vi "Read X-Axis.vi"(6 "Maximum Time (10000 ms)":u32=10000, 8 "error in (no error)":errorcluster, 9 "Select Trace (1: 1)":u16(ring)=1 items=["1"=1, "2"=2, "3"=3, "4"=4, "5"=5, "6"=6, "7"=7, "8"=8], 10 "Measurement Type (6: Phase Noise)":u16(ring)=6 items=["AM Noise"=1, "Baseband Noise"=2, "Freq/Power"=3, "Spectrum"=4, "Transient"=5, "Phase Noise"=6, "User"=7], 11 "VISA resource name":refnum<visa-resource-name>) -> (0 "error out":errorcluster, 2 "Measurements":dbl[](array[numeric]) format="%^#_9g", 3 "VISA resource name out":refnum<visa-resource-name>)   [LabVIEW 2011, in "Agilent E5052X.lvlib"]
doc: "Reads X-axis trace data from the instrument."
uses:
  Agilent E5052X.lvlib
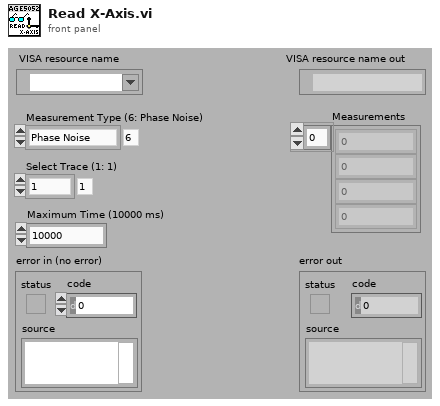
[diagram p1: front panel]
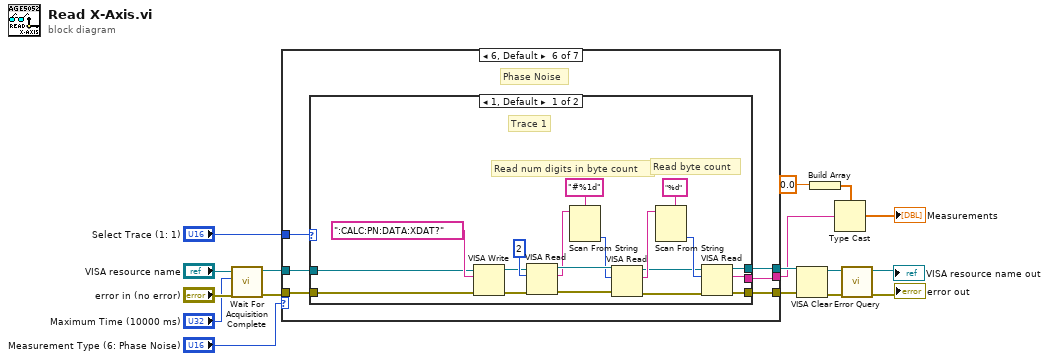
[diagram p0: block diagram]
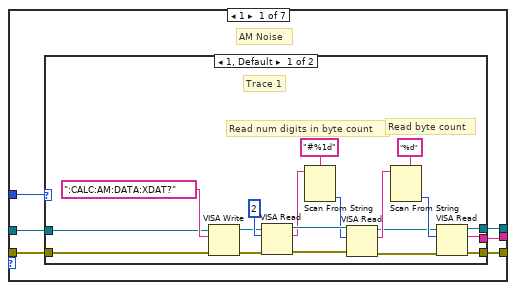
[diagram p2: hidden frame]
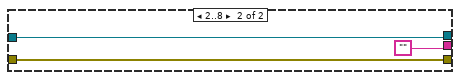
[diagram p3: hidden frame]
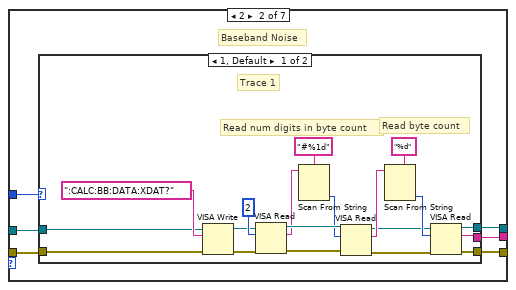
[diagram p4: hidden frame]
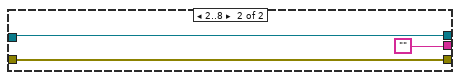
[diagram p5: hidden frame]
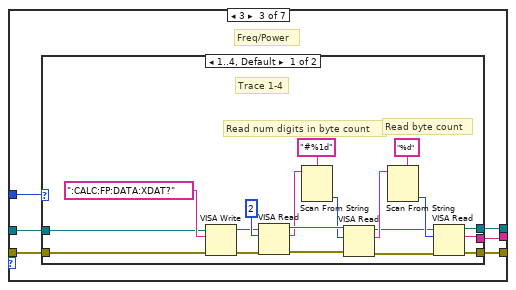
[diagram p6: hidden frame]
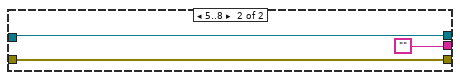
[diagram p7: hidden frame]
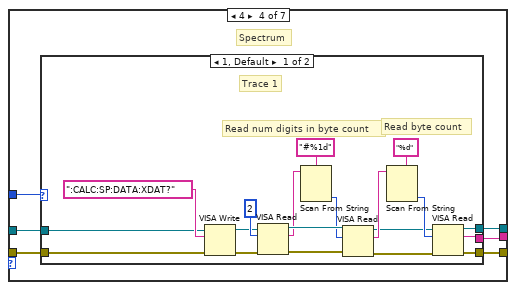
[diagram p8: hidden frame]
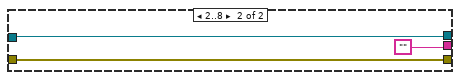
[diagram p9: hidden frame]
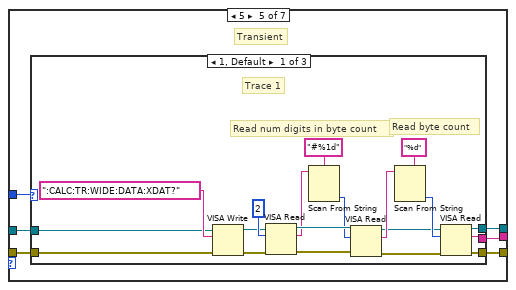
[diagram p10: hidden frame]
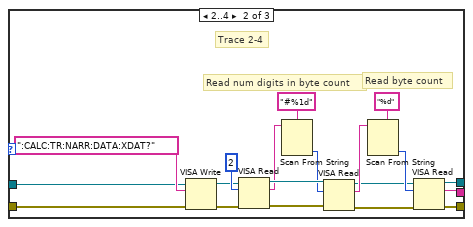
[diagram p11: hidden frame]
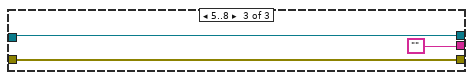
[diagram p12: hidden frame]
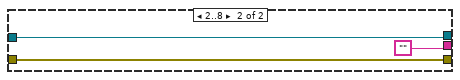
[diagram p13: hidden frame]
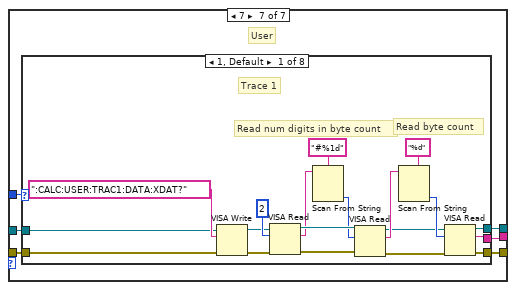
[diagram p14: hidden frame]
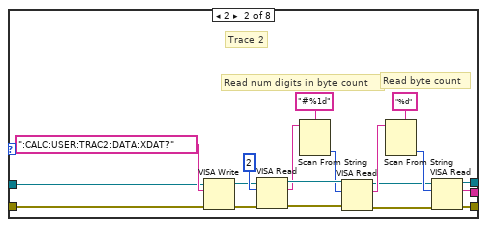
[diagram p15: hidden frame]
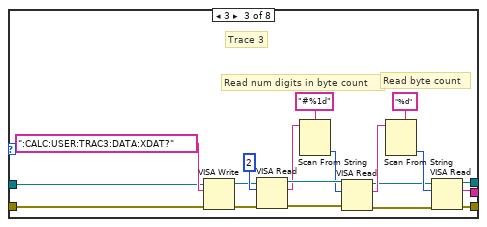
[diagram p16: hidden frame]
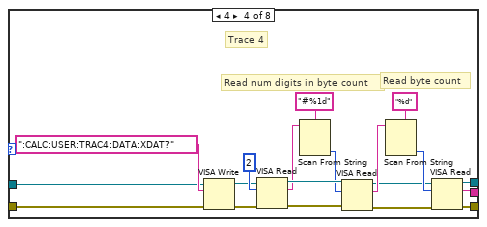
[diagram p17: hidden frame]
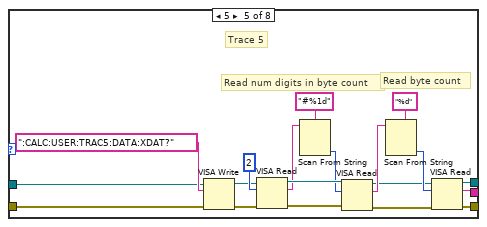
[diagram p18: hidden frame]
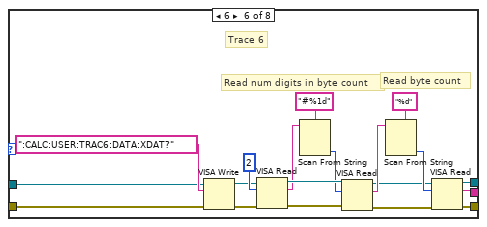
[diagram p19: hidden frame]
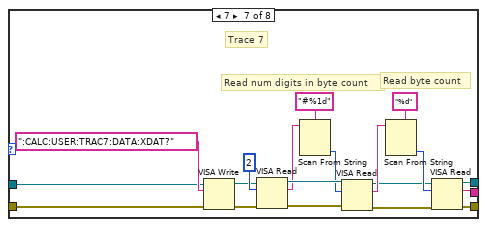
[diagram p20: hidden frame]
diagram:
  n1 = call "Wait For Acquisition Complete.vi"("error in (no error)"="error in (no error)", "Maximum Time (10000)"="Maximum Time (10000 ms)", "VISA resource name"="VISA resource name") -> ("error out"=w11:errorcluster, "VISA resource name out"=w10:refnum<visa-resource-name>)  [unwired: 7 in]
  n2 = case shown="6, Default" "Measurement Type (6: Phase Noise)" {
    tunnel: w10 -> [w22 w50 w78 w106 w134 w181 w209]
    tunnel: w11 -> [w21 w49 w77 w105 w133 w180 w208]
    tunnel: "Select Trace (1: 1)" -> [w23 w51 w79 w107 w135 w182 w210]
    tunnel: [w20 w48 w76 w104 w132 w179 w207] -> w13
    tunnel: [w19 w46 w74 w102 w130 w177 w205] -> w12
    tunnel: [w18 w47 w75 w103 w131 w178 w206] -> w2
    frame 1 {
      # "AM Noise"
      n3 = case shown="1, Default" w23 {
        tunnel: w22 -> [w41 w45]
        tunnel: w21 -> [w40 w44]
        tunnel: [w26 w45] -> w20
        tunnel: [w25 w44] -> w19
        tunnel: [w24 ""] -> w18
        frame 1, Default {
          # "Read num digits in byte count"
          # "Read byte count"
          # "Trace 1"
          n4 = VISA Write(VISA resource name=w41, write buffer=":CALC:AM:DATA:XDAT?" ("format string"), error in (no error)=w40) -> (VISA resource name out=w30:refnum<visa-resource-name>, error out=w29:errorcluster)  [unwired: 1 out]
          n5 = VISA Read(VISA resource name=w30, byte count=u32 2, error in (no error)=w29) -> (VISA resource name out=w36:refnum<visa-resource-name>, read buffer=w32:string, error out=w37:errorcluster)  [unwired: 1 out]
          n6 = Scan From String(format string="#%1d", input string=w32) -> (output 1=w35:i32)  [unwired: 3 in, 3 out]
          n7 = VISA Read(VISA resource name=w36, byte count=w35, error in (no error)=w37) -> (VISA resource name out=w28:refnum<visa-resource-name>, read buffer=w34:string, error out=w27:errorcluster)  [unwired: 1 out]
          n8 = Scan From String(format string="%d", input string=w34) -> (output 1=w31:i32)  [unwired: 3 in, 3 out]
          n9 = VISA Read(VISA resource name=w28, byte count=w31, error in (no error)=w27) -> (VISA resource name out=w26:refnum<visa-resource-name>, read buffer=w24:string, error out=w25:errorcluster)  [unwired: 1 out]
        }
        frame 2..8 {
        }
      }
    }
    frame 2 {
      # "Baseband Noise"
      n10 = case shown="1, Default" w51 {
        tunnel: w50 -> [w69 w73]
        tunnel: w49 -> [w68 w72]
        tunnel: [w54 w73] -> w48
        tunnel: [w53 w72] -> w46
        tunnel: [w52 ""] -> w47
        frame 1, Default {
          # "Read num digits in byte count"
          # "Read byte count"
          # "Trace 1"
          n11 = VISA Write(VISA resource name=w69, write buffer=":CALC:BB:DATA:XDAT?" ("format string"), error in (no error)=w68) -> (VISA resource name out=w58:refnum<visa-resource-name>, error out=w57:errorcluster)  [unwired: 1 out]
          n12 = VISA Read(VISA resource name=w58, byte count=u32 2, error in (no error)=w57) -> (VISA resource name out=w64:refnum<visa-resource-name>, read buffer=w60:string, error out=w65:errorcluster)  [unwired: 1 out]
          n13 = Scan From String(format string="#%1d", input string=w60) -> (output 1=w63:i32)  [unwired: 3 in, 3 out]
          n14 = VISA Read(VISA resource name=w64, byte count=w63, error in (no error)=w65) -> (VISA resource name out=w56:refnum<visa-resource-name>, read buffer=w62:string, error out=w55:errorcluster)  [unwired: 1 out]
          n15 = Scan From String(format string="%d", input string=w62) -> (output 1=w59:i32)  [unwired: 3 in, 3 out]
          n16 = VISA Read(VISA resource name=w56, byte count=w59, error in (no error)=w55) -> (VISA resource name out=w54:refnum<visa-resource-name>, read buffer=w52:string, error out=w53:errorcluster)  [unwired: 1 out]
        }
        frame 2..8 {
        }
      }
    }
    frame 3 {
      # "Freq/Power"
      n17 = case shown="1..4, Default" w79 {
        tunnel: w78 -> [w97 w101]
        tunnel: w77 -> [w96 w100]
        tunnel: [w82 w101] -> w76
        tunnel: [w81 w100] -> w74
        tunnel: [w80 ""] -> w75
        frame 1..4, Default {
          # "Trace 1-4"
          # "Read num digits in byte count"
          # "Read byte count"
          n18 = VISA Write(VISA resource name=w97, write buffer=":CALC:FP:DATA:XDAT?" ("format string"), error in (no error)=w96) -> (VISA resource name out=w86:refnum<visa-resource-name>, error out=w85:errorcluster)  [unwired: 1 out]
          n19 = VISA Read(VISA resource name=w86, byte count=u32 2, error in (no error)=w85) -> (VISA resource name out=w92:refnum<visa-resource-name>, read buffer=w88:string, error out=w93:errorcluster)  [unwired: 1 out]
          n20 = Scan From String(format string="#%1d", input string=w88) -> (output 1=w91:i32)  [unwired: 3 in, 3 out]
          n21 = VISA Read(VISA resource name=w92, byte count=w91, error in (no error)=w93) -> (VISA resource name out=w84:refnum<visa-resource-name>, read buffer=w90:string, error out=w83:errorcluster)  [unwired: 1 out]
          n22 = Scan From String(format string="%d", input string=w90) -> (output 1=w87:i32)  [unwired: 3 in, 3 out]
          n23 = VISA Read(VISA resource name=w84, byte count=w87, error in (no error)=w83) -> (VISA resource name out=w82:refnum<visa-resource-name>, read buffer=w80:string, error out=w81:errorcluster)  [unwired: 1 out]
        }
        frame 5..8 {
        }
      }
    }
    frame 4 {
      # "Spectrum"
      n24 = case shown="1, Default" w107 {
        tunnel: w106 -> [w125 w127]
        tunnel: w105 -> [w124 w129]
        tunnel: [w110 w127] -> w104
        tunnel: [w109 w129] -> w102
        tunnel: [w108 ""] -> w103
        frame 1, Default {
          # "Read num digits in byte count"
          # "Read byte count"
          # "Trace 1"
          n25 = VISA Write(VISA resource name=w125, write buffer=":CALC:SP:DATA:XDAT?" ("format string"), error in (no error)=w124) -> (VISA resource name out=w114:refnum<visa-resource-name>, error out=w113:errorcluster)  [unwired: 1 out]
          n26 = VISA Read(VISA resource name=w114, byte count=u32 2, error in (no error)=w113) -> (VISA resource name out=w120:refnum<visa-resource-name>, read buffer=w116:string, error out=w121:errorcluster)  [unwired: 1 out]
          n27 = Scan From String(format string="#%1d", input string=w116) -> (output 1=w119:i32)  [unwired: 3 in, 3 out]
          n28 = VISA Read(VISA resource name=w120, byte count=w119, error in (no error)=w121) -> (VISA resource name out=w112:refnum<visa-resource-name>, read buffer=w118:string, error out=w111:errorcluster)  [unwired: 1 out]
          n29 = Scan From String(format string="%d", input string=w118) -> (output 1=w115:i32)  [unwired: 3 in, 3 out]
          n30 = VISA Read(VISA resource name=w112, byte count=w115, error in (no error)=w111) -> (VISA resource name out=w110:refnum<visa-resource-name>, read buffer=w108:string, error out=w109:errorcluster)  [unwired: 1 out]
        }
        frame 2..8 {
        }
      }
    }
    frame 5 {
      # "Transient"
      n31 = case shown="1, Default" w135 {
        tunnel: w134 -> [w140 w172 w176]
        tunnel: w133 -> [w139 w171 w175]
        tunnel: [w138 w157 w176] -> w132
        tunnel: [w136 w156 w175] -> w130
        tunnel: [w137 w155 ""] -> w131
        frame 1, Default {
          # "Trace 1"
          # "Read num digits in byte count"
          # "Read byte count"
          n32 = VISA Write(VISA resource name=w140, write buffer=":CALC:TR:WIDE:DATA:XDAT?" ("format string"), error in (no error)=w139) -> (VISA resource name out=w144:refnum<visa-resource-name>, error out=w143:errorcluster)  [unwired: 1 out]
          n33 = VISA Read(VISA resource name=w144, byte count=u32 2, error in (no error)=w143) -> (VISA resource name out=w150:refnum<visa-resource-name>, read buffer=w146:string, error out=w151:errorcluster)  [unwired: 1 out]
          n34 = Scan From String(format string="#%1d", input string=w146) -> (output 1=w149:i32)  [unwired: 3 in, 3 out]
          n35 = VISA Read(VISA resource name=w150, byte count=w149, error in (no error)=w151) -> (VISA resource name out=w142:refnum<visa-resource-name>, read buffer=w148:string, error out=w141:errorcluster)  [unwired: 1 out]
          n36 = Scan From String(format string="%d", input string=w148) -> (output 1=w145:i32)  [unwired: 3 in, 3 out]
          n37 = VISA Read(VISA resource name=w142, byte count=w145, error in (no error)=w141) -> (VISA resource name out=w138:refnum<visa-resource-name>, read buffer=w137:string, error out=w136:errorcluster)  [unwired: 1 out]
        }
        frame 2..4 {
          # "Trace 2-4"
          # "Read num digits in byte count"
          # "Read byte count"
          n38 = VISA Write(VISA resource name=w172, write buffer=":CALC:TR:NARR:DATA:XDAT?" ("format string"), error in (no error)=w171) -> (VISA resource name out=w161:refnum<visa-resource-name>, error out=w160:errorcluster)  [unwired: 1 out]
          n39 = VISA Read(VISA resource name=w161, byte count=u32 2, error in (no error)=w160) -> (VISA resource name out=w167:refnum<visa-resource-name>, read buffer=w163:string, error out=w168:errorcluster)  [unwired: 1 out]
          n40 = Scan From String(format string="#%1d", input string=w163) -> (output 1=w166:i32)  [unwired: 3 in, 3 out]
          n41 = VISA Read(VISA resource name=w167, byte count=w166, error in (no error)=w168) -> (VISA resource name out=w159:refnum<visa-resource-name>, read buffer=w165:string, error out=w158:errorcluster)  [unwired: 1 out]
          n42 = Scan From String(format string="%d", input string=w165) -> (output 1=w162:i32)  [unwired: 3 in, 3 out]
          n43 = VISA Read(VISA resource name=w159, byte count=w162, error in (no error)=w158) -> (VISA resource name out=w157:refnum<visa-resource-name>, read buffer=w155:string, error out=w156:errorcluster)  [unwired: 1 out]
        }
        frame 5..8 {
        }
      }
    }
    frame 6, Default {
      # "Phase Noise"
      n44 = case shown="1, Default" w182 {
        tunnel: w181 -> [w200 w204]
        tunnel: w180 -> [w199 w203]
        tunnel: [w185 w204] -> w179
        tunnel: [w184 w203] -> w177
        tunnel: [w183 ""] -> w178
        frame 1, Default {
          # "Read num digits in byte count"
          # "Read byte count"
          # "Trace 1"
          n45 = VISA Write(VISA resource name=w200, write buffer=":CALC:PN:DATA:XDAT?" ("format string"), error in (no error)=w199) -> (VISA resource name out=w189:refnum<visa-resource-name>, error out=w188:errorcluster)  [unwired: 1 out]
          n46 = VISA Read(VISA resource name=w189, byte count=u32 2, error in (no error)=w188) -> (VISA resource name out=w195:refnum<visa-resource-name>, read buffer=w191:string, error out=w196:errorcluster)  [unwired: 1 out]
          n47 = Scan From String(format string="#%1d", input string=w191) -> (output 1=w194:i32)  [unwired: 3 in, 3 out]
          n48 = VISA Read(VISA resource name=w195, byte count=w194, error in (no error)=w196) -> (VISA resource name out=w187:refnum<visa-resource-name>, read buffer=w193:string, error out=w186:errorcluster)  [unwired: 1 out]
          n49 = Scan From String(format string="%d", input string=w193) -> (output 1=w190:i32)  [unwired: 3 in, 3 out]
          n50 = VISA Read(VISA resource name=w187, byte count=w190, error in (no error)=w186) -> (VISA resource name out=w185:refnum<visa-resource-name>, read buffer=w183:string, error out=w184:errorcluster)  [unwired: 1 out]
        }
        frame 2..8 {
        }
      }
    }
    frame 7 {
      # "User"
      n51 = case shown="1, Default" w210 {
        tunnel: w209 -> [w228 w247 w266 w285 w304 w323 w342 w361]
        tunnel: w208 -> [w227 w246 w265 w284 w303 w322 w341 w360]
        tunnel: [w213 w232 w251 w270 w289 w308 w327 w346] -> w207
        tunnel: [w212 w231 w250 w269 w288 w307 w326 w345] -> w205
        tunnel: [w211 w230 w249 w268 w287 w306 w325 w344] -> w206
        frame 1, Default {
          # "Trace 1"
          # "Read num digits in byte count"
          # "Read byte count"
          n52 = VISA Write(VISA resource name=w228, write buffer=":CALC:USER:TRAC1:DATA:XDAT?" ("format string"), error in (no error)=w227) -> (VISA resource name out=w217:refnum<visa-resource-name>, error out=w216:errorcluster)  [unwired: 1 out]
          n53 = VISA Read(VISA resource name=w217, byte count=u32 2, error in (no error)=w216) -> (VISA resource name out=w223:refnum<visa-resource-name>, read buffer=w219:string, error out=w224:errorcluster)  [unwired: 1 out]
          n54 = Scan From String(format string="#%1d", input string=w219) -> (output 1=w222:i32)  [unwired: 3 in, 3 out]
          n55 = VISA Read(VISA resource name=w223, byte count=w222, error in (no error)=w224) -> (VISA resource name out=w215:refnum<visa-resource-name>, read buffer=w221:string, error out=w214:errorcluster)  [unwired: 1 out]
          n56 = Scan From String(format string="%d", input string=w221) -> (output 1=w218:i32)  [unwired: 3 in, 3 out]
          n57 = VISA Read(VISA resource name=w215, byte count=w218, error in (no error)=w214) -> (VISA resource name out=w213:refnum<visa-resource-name>, read buffer=w211:string, error out=w212:errorcluster)  [unwired: 1 out]
        }
        frame 2 {
          # "Trace 2"
          # "Read num digits in byte count"
          # "Read byte count"
          n58 = VISA Write(VISA resource name=w247, write buffer=":CALC:USER:TRAC2:DATA:XDAT?" ("format string"), error in (no error)=w246) -> (VISA resource name out=w236:refnum<visa-resource-name>, error out=w235:errorcluster)  [unwired: 1 out]
          n59 = VISA Read(VISA resource name=w236, byte count=u32 2, error in (no error)=w235) -> (VISA resource name out=w242:refnum<visa-resource-name>, read buffer=w238:string, error out=w243:errorcluster)  [unwired: 1 out]
          n60 = Scan From String(format string="#%1d", input string=w238) -> (output 1=w241:i32)  [unwired: 3 in, 3 out]
          n61 = VISA Read(VISA resource name=w242, byte count=w241, error in (no error)=w243) -> (VISA resource name out=w234:refnum<visa-resource-name>, read buffer=w240:string, error out=w233:errorcluster)  [unwired: 1 out]
          n62 = Scan From String(format string="%d", input string=w240) -> (output 1=w237:i32)  [unwired: 3 in, 3 out]
          n63 = VISA Read(VISA resource name=w234, byte count=w237, error in (no error)=w233) -> (VISA resource name out=w232:refnum<visa-resource-name>, read buffer=w230:string, error out=w231:errorcluster)  [unwired: 1 out]
        }
        frame 3 {
          # "Trace 3"
          # "Read num digits in byte count"
          # "Read byte count"
          n64 = VISA Write(VISA resource name=w266, write buffer=":CALC:USER:TRAC3:DATA:XDAT?" ("format string"), error in (no error)=w265) -> (VISA resource name out=w255:refnum<visa-resource-name>, error out=w254:errorcluster)  [unwired: 1 out]
          n65 = VISA Read(VISA resource name=w255, byte count=u32 2, error in (no error)=w254) -> (VISA resource name out=w261:refnum<visa-resource-name>, read buffer=w257:string, error out=w262:errorcluster)  [unwired: 1 out]
          n66 = Scan From String(format string="#%1d", input string=w257) -> (output 1=w260:i32)  [unwired: 3 in, 3 out]
          n67 = VISA Read(VISA resource name=w261, byte count=w260, error in (no error)=w262) -> (VISA resource name out=w253:refnum<visa-resource-name>, read buffer=w259:string, error out=w252:errorcluster)  [unwired: 1 out]
          n68 = Scan From String(format string="%d", input string=w259) -> (output 1=w256:i32)  [unwired: 3 in, 3 out]
          n69 = VISA Read(VISA resource name=w253, byte count=w256, error in (no error)=w252) -> (VISA resource name out=w251:refnum<visa-resource-name>, read buffer=w249:string, error out=w250:errorcluster)  [unwired: 1 out]
        }
        frame 4 {
          # "Trace 4"
          # "Read num digits in byte count"
          # "Read byte count"
          n70 = VISA Write(VISA resource name=w285, write buffer=":CALC:USER:TRAC4:DATA:XDAT?" ("format string"), error in (no error)=w284) -> (VISA resource name out=w274:refnum<visa-resource-name>, error out=w273:errorcluster)  [unwired: 1 out]
          n71 = VISA Read(VISA resource name=w274, byte count=u32 2, error in (no error)=w273) -> (VISA resource name out=w280:refnum<visa-resource-name>, read buffer=w276:string, error out=w281:errorcluster)  [unwired: 1 out]
          n72 = Scan From String(format string="#%1d", input string=w276) -> (output 1=w279:i32)  [unwired: 3 in, 3 out]
          n73 = VISA Read(VISA resource name=w280, byte count=w279, error in (no error)=w281) -> (VISA resource name out=w272:refnum<visa-resource-name>, read buffer=w278:string, error out=w271:errorcluster)  [unwired: 1 out]
          n74 = Scan From String(format string="%d", input string=w278) -> (output 1=w275:i32)  [unwired: 3 in, 3 out]
          n75 = VISA Read(VISA resource name=w272, byte count=w275, error in (no error)=w271) -> (VISA resource name out=w270:refnum<visa-resource-name>, read buffer=w268:string, error out=w269:errorcluster)  [unwired: 1 out]
        }
        frame 5 {
          # "Trace 5"
          # "Read num digits in byte count"
          # "Read byte count"
          n76 = VISA Write(VISA resource name=w304, write buffer=":CALC:USER:TRAC5:DATA:XDAT?" ("format string"), error in (no error)=w303) -> (VISA resource name out=w293:refnum<visa-resource-name>, error out=w292:errorcluster)  [unwired: 1 out]
          n77 = VISA Read(VISA resource name=w293, byte count=u32 2, error in (no error)=w292) -> (VISA resource name out=w299:refnum<visa-resource-name>, read buffer=w295:string, error out=w300:errorcluster)  [unwired: 1 out]
          n78 = Scan From String(format string="#%1d", input string=w295) -> (output 1=w298:i32)  [unwired: 3 in, 3 out]
          n79 = VISA Read(VISA resource name=w299, byte count=w298, error in (no error)=w300) -> (VISA resource name out=w291:refnum<visa-resource-name>, read buffer=w297:string, error out=w290:errorcluster)  [unwired: 1 out]
          n80 = Scan From String(format string="%d", input string=w297) -> (output 1=w294:i32)  [unwired: 3 in, 3 out]
          n81 = VISA Read(VISA resource name=w291, byte count=w294, error in (no error)=w290) -> (VISA resource name out=w289:refnum<visa-resource-name>, read buffer=w287:string, error out=w288:errorcluster)  [unwired: 1 out]
        }
        frame 6 {
          # "Trace 6"
          # "Read num digits in byte count"
          # "Read byte count"
          n82 = VISA Write(VISA resource name=w323, write buffer=":CALC:USER:TRAC6:DATA:XDAT?" ("format string"), error in (no error)=w322) -> (VISA resource name out=w312:refnum<visa-resource-name>, error out=w311:errorcluster)  [unwired: 1 out]
          n83 = VISA Read(VISA resource name=w312, byte count=u32 2, error in (no error)=w311) -> (VISA resource name out=w318:refnum<visa-resource-name>, read buffer=w314:string, error out=w319:errorcluster)  [unwired: 1 out]
          n84 = Scan From String(format string="#%1d", input string=w314) -> (output 1=w317:i32)  [unwired: 3 in, 3 out]
          n85 = VISA Read(VISA resource name=w318, byte count=w317, error in (no error)=w319) -> (VISA resource name out=w310:refnum<visa-resource-name>, read buffer=w316:string, error out=w309:errorcluster)  [unwired: 1 out]
          n86 = Scan From String(format string="%d", input string=w316) -> (output 1=w313:i32)  [unwired: 3 in, 3 out]
          n87 = VISA Read(VISA resource name=w310, byte count=w313, error in (no error)=w309) -> (VISA resource name out=w308:refnum<visa-resource-name>, read buffer=w306:string, error out=w307:errorcluster)  [unwired: 1 out]
        }
        frame 7 {
          # "Trace 7"
          # "Read num digits in byte count"
          # "Read byte count"
          n88 = VISA Write(VISA resource name=w342, write buffer=":CALC:USER:TRAC7:DATA:XDAT?" ("format string"), error in (no error)=w341) -> (VISA resource name out=w331:refnum<visa-resource-name>, error out=w330:errorcluster)  [unwired: 1 out]
          n89 = VISA Read(VISA resource name=w331, byte count=u32 2, error in (no error)=w330) -> (VISA resource name out=w337:refnum<visa-resource-name>, read buffer=w333:string, error out=w338:errorcluster)  [unwired: 1 out]
          n90 = Scan From String(format string="#%1d", input string=w333) -> (output 1=w336:i32)  [unwired: 3 in, 3 out]
          n91 = VISA Read(VISA resource name=w337, byte count=w336, error in (no error)=w338) -> (VISA resource name out=w329:refnum<visa-resource-name>, read buffer=w335:string, error out=w328:errorcluster)  [unwired: 1 out]
          n92 = Scan From String(format string="%d", input string=w335) -> (output 1=w332:i32)  [unwired: 3 in, 3 out]
          n93 = VISA Read(VISA resource name=w329, byte count=w332, error in (no error)=w328) -> (VISA resource name out=w327:refnum<visa-resource-name>, read buffer=w325:string, error out=w326:errorcluster)  [unwired: 1 out]
        }
        frame 8 {
          # "Trace 8"
          # "Read num digits in byte count"
          # "Read byte count"
          n94 = VISA Write(VISA resource name=w361, write buffer=":CALC:USER:TRAC8:DATA:XDAT?" ("format string"), error in (no error)=w360) -> (VISA resource name out=w350:refnum<visa-resource-name>, error out=w349:errorcluster)  [unwired: 1 out]
          n95 = VISA Read(VISA resource name=w350, byte count=u32 2, error in (no error)=w349) -> (VISA resource name out=w356:refnum<visa-resource-name>, read buffer=w352:string, error out=w357:errorcluster)  [unwired: 1 out]
          n96 = Scan From String(format string="#%1d", input string=w352) -> (output 1=w355:i32)  [unwired: 3 in, 3 out]
          n97 = VISA Read(VISA resource name=w356, byte count=w355, error in (no error)=w357) -> (VISA resource name out=w348:refnum<visa-resource-name>, read buffer=w354:string, error out=w347:errorcluster)  [unwired: 1 out]
          n98 = Scan From String(format string="%d", input string=w354) -> (output 1=w351:i32)  [unwired: 3 in, 3 out]
          n99 = VISA Read(VISA resource name=w348, byte count=w351, error in (no error)=w347) -> (VISA resource name out=w346:refnum<visa-resource-name>, read buffer=w344:string, error out=w345:errorcluster)  [unwired: 1 out]
        }
      }
    }
  }
  n100 = VISA Clear(VISA resource name=w13, error in (no error)=w12) -> (VISA resource name out=w6:refnum<visa-resource-name>, error out=w5:errorcluster)
  n101 = Build Array(sgl 0.0) -> (w3:sgl[])
  n102 = Type Cast(type=w3, x=w2) -> (*(type *) &x=→"Measurements":sgl[])
  n103 = call "Error Query.vi"("error in (no error)"=w5, "VISA resource name"=w6) -> ("error out"=→"error out":errorcluster, "VISA resource name out"=→"VISA resource name out":refnum<visa-resource-name>)  [unwired: 6 in, 2 out]
